vi "LVClass_Pupil ctor from txt file.vi"(0 "Pupil in":refnum<class "Pupil.lvclass">, 5 "file path txt":path, 11 "error in (no error)":errorcluster) -> (4 "Pupil out":refnum<class "Pupil.lvclass">, 15 "error out":errorcluster)   [LabVIEW 2020, in "Pupil.lvclass"]
doc: "Circular Pupil constructor from dimensions, steps and circle shape.\n\n--------------------------------------------------------------------------------\n\n<B>PupilIn </B> : Constant Pointer to Pupil object.\n<B>PupilOut </B> : Constant Pointer to Pupil object.\n<B>step </B> : Step x and y between the subpupils (um).\n<B>dimensions </B> : Pupil array dimensions (width, height).\n<B>center </B> : Center of the circle shape (um).\n<B>radius </B> : Radius of the circle shape (um).\n<B>ErrorIn </B> : Error\n<B>ErrorOut </B> : Error\n\n--------------------------------------------------------------------------------"
uses:
  Pupil.lvclass
  General dimensions definition.ctl
  Point2D.ctl
  Point2Df.ctl
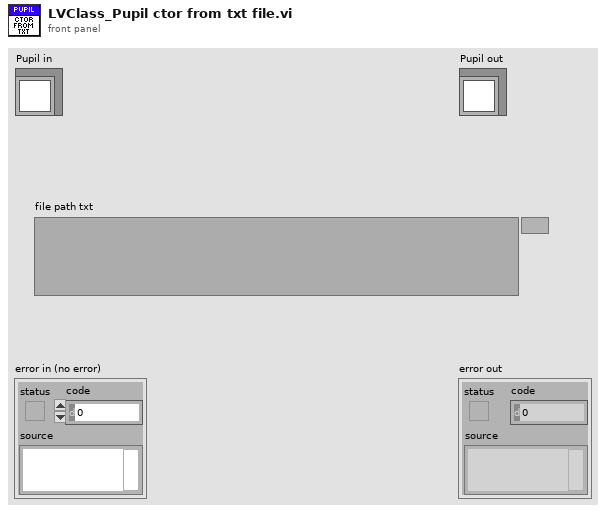
[diagram p1: front panel]
types:
  T1 = typedef "Point2Df.ctl" = cluster{"X":sgl, "Y":sgl}
  T2 = typedef "General dimensions definition.ctl" = cluster{"Size":T3, "Step":T1}
  T3 = typedef "Point2D.ctl" = cluster{"X":u32, "Y":u32}
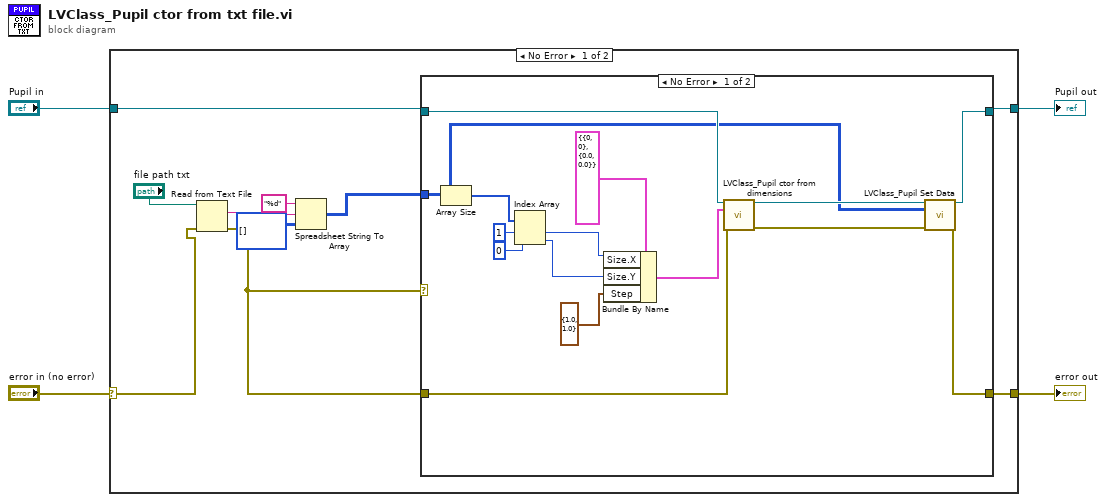
[diagram p0: block diagram]
diagram:
  n1 = case shown="No Error" "error in (no error)" {
    selector: "error in (no error)" -> [w7 w33]
    tunnel: [w13 w33] -> w3
    tunnel: [w12 w32] -> w1
    tunnel: "Pupil in" -> [w14 w32]
    frame No Error {
      n2 = Read from Text File(file (use dialog)="file path txt", error in=w7) -> (text=w6:string, error out=w5:errorcluster)  [unwired: 2 in, 2 out]
      n3 = Spreadsheet String To Array(format string="%d", spreadsheet string=w6, array type (2D Dbl)=u8[][] []) -> (array=w9:u8[][])  [unwired: 1 in]
      n4 = case shown="No Error" w5 {
        tunnel: w14 -> [w21 w31]
        tunnel: w5 -> [w20 w30]
        tunnel: w9 -> [w15 _]
        tunnel: [w18 w30] -> w13
        tunnel: [w16 w31] -> w12
        frame No Error {
          n5 = Array Size(array=w15) -> (size(s)=w28:i32[])
          n6 = Index Array(array=w28, index #1=1 ("index"), index #2=0 ("index")) -> (element #1=w25:i32, element #2=w24:i32)
          n7 = Bundle By Name(cluster=T2 {"Size"={"X"=0, "Y"=0}, "Step"={"X"=0.0, "Y"=0.0}} ("Dimensions_µm"), "Size.X"=w25, "Size.Y"=w24, "Step"=T1 {"X"=1.0, "Y"=1.0}) -> (w22:T2)
          n8 = call "LVClass_Pupil ctor from dimensions.vi"("Pupil in"=w21, "Dimensions_um"=w22, "error in (no error)"=w20) -> ("Pupil out"=w17:refnum<class "Pupil.lvclass">, "error out"=w19:errorcluster)  [unwired: 11 in]
          n9 = call "LVClass_Pupil Set Data.vi"("Pupil in"=w17, "Data"=w15, "error in (no error)"=w19) -> ("Pupil out"=w16:refnum<class "Pupil.lvclass">, "error out"=w18:errorcluster)  [unwired: 11 in]
        }
        frame Error {
        }
      }
    }
    frame Error {
    }
  }
  "error out" <- w3
  "Pupil out" <- w1
